vi "S30c_dll F33.vi"(2 "Config Byte":u8, 4 "error in":errorcluster, 6 "Nr.":u8, 7 "Dev Addr":u8=250) -> (0 "error out":errorcluster, 1 "Org. Config Byte":u8)   [LabVIEW 2014, in "K_S30c_dll.lvlib"]
uses:
  K_S30c_dll.lvlib
  s30c.dll
panel:
  # "Function 33: Write configuration \nWarning!!\n\nPlease be careful, using this function! \nWrong configuration changes the function of the device! \nMake sure that you save first the origignal configuration with F32.\n\nusing s30c.dll\nKeller AG für Druckmesstechnik, 29.5.08 b.v."
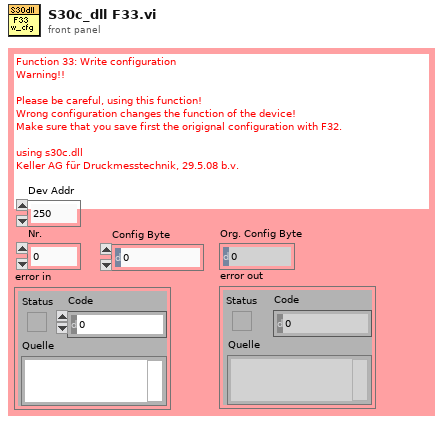
[diagram p1: front panel]
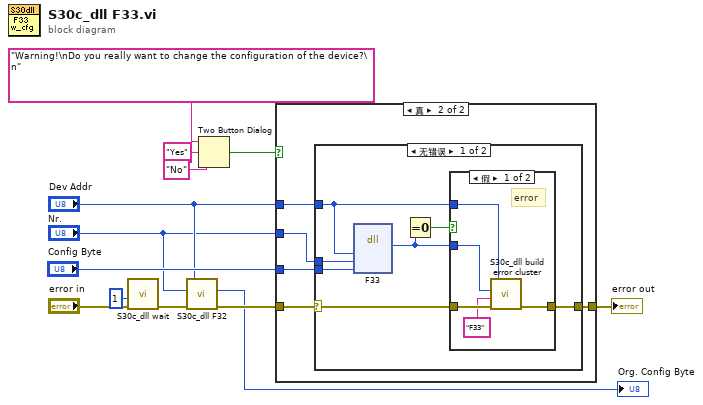
[diagram p0: block diagram]
diagram:
  n1 = call "S30c_dll wait.vi"("error in (no error)"="error in", "Time [ms]"=u32 1) -> ("error out"=w2:errorcluster)  [unwired: 5 in]
  n2 = call "S30c_dll F32.vi"("error in"=w2, "Nr."="Nr.", "Dev Addr"="Dev Addr") -> ("error out"=w7:errorcluster, "Config Byte"=→"Org. Config Byte":u8)  [unwired: 3 in]
  n3 = Two Button Dialog(message="Warning!\nDo you really want to change the configuration of the device?\n" ("Nachricht"), 1:"No" ("F-Schaltflächenname (\"Abbrechen\")"), 2:"Yes" ("T-Schaltflächenname (\"OK\")")) -> (T button?=w8:bool)
  n4 = case shown="真" w8 {
    tunnel: "Dev Addr" -> [_ w19]
    tunnel: w7 -> [w14 w18]
    tunnel: "Nr." -> [_ w17]
    tunnel: [w14 w16] -> w13
    tunnel: "Config Byte" -> [_ w15]
    frame False {
    }
    frame True {
      n5 = case shown="无错误" w18 {
        selector: w18 -> [w24 w33]
        tunnel: [w25 w33] -> w16
        tunnel: w19 -> [w23 _]
        tunnel: w17 -> [w22 _]
        tunnel: w15 -> [w21 _]
        frame No Error {
          n6 = dll-call lib="PTH2Labs EworkSINOPEC北控自动相渗software2.08.5_dlls30c.dll" fn="F33"("DevAddr"=w23, "Coeff No"=w22, "Coeff"=w21) -> (w20:i16)  [unwired: 6 in, 2 out]
          n7 = Equal To 0?(x=w20) -> (x = 0?=w26:bool)
          n8 = case shown="假" w26 {
            tunnel: w24 -> [w31 w32]
            tunnel: [w30 w32] -> w25
            tunnel: w23 -> [w28 _]
            tunnel: w20 -> [w27 _]
            frame False {
              # "error"
              n9 = call "S30c_dll build error cluster.vi"("error in"=w31, "error Text"="F33", "error code"=w27, "Dev Addr"=w28) -> ("error out"=w30:errorcluster)  [unwired: 3 in]
            }
            frame True {
            }
          }
        }
        frame Error {
        }
      }
    }
  }
  "error out" <- w13
